vi "Robot Global Data.vi"() -> ()   [LabVIEW 2019]
doc: "This global VI can contain as many global variables as you need. Place a control on the panel, give it a good name. To read or write to it from a VI, drag the icon to the diagram of that VI. You can also drag from the project. Click on the node to change which global you access. You shouldn't have multiple locations writing to a global or it will cause a race-condition."
uses:
  <vilib>/Rock Robotics/WPI/Camera/WPI_CameraImageSize.ctl
  <vilib>/Rock Robotics/WPI/DriverStation/WPI_DriverStationRobotMode2.ctl
panel:
  out "Winch Speed":dbl
  in  "Winch":bool
  in  "OC_Winch":bool
  out "Flywheel Position":dbl
  out "Turret Type":string
  out "Turret Swiv Position":dbl
  out "Flywheel 2 Velocity":dbl
  out "Flywheel 1 Velocity":dbl
  in  "Elevator Allowed":bool
  out "Turret Pos":dbl
  out "Brake Climb":bool
  out "OC_Turret Zero":bool
  in  "Required Flywheel Speed":dbl
  out "Flywheel Speed":dbl
  out "Flywheels":bool
  out "OC_Flywheels On":bool
  out "OC_Flywheels Off":bool
  out "Fire":bool
  out "OC_Fire":bool
  in  "Turret Semi":bool
  out "OC_Turret Semi":bool
  in  "Ball Taken":bool
  out "Tower Feed On":bool
  out "Cell Counter":dbl
  in  "Tower Auto":bool
  out "OC_Tower Auto":bool
  in  "Man Tower Feed":bool
  out "OC_Man Tower Feed":bool
  out "Tower LS On":bool
  in  "Zoom In":bool
  out "OC_Lime Zoom":bool
  out "VP On":bool
  out "OC_VP Off":bool
  out "OC_VP On":bool
  out "Shooter Feed On":bool
  out "OC_Shooter Feed":bool
  out "OC_Tower Unjam":bool
  in  "Tower Unjam":bool
  out "Shooter Feed":dbl
  out "Tower Storage":dbl
  out "Tower Feed":dbl
  out "Turret Vert Value":dbl
  in  "Intake Unjam":bool
  out "DC_Intake Unjam":bool
  out "Intake Speed":dbl
  out "DC_Intake Off":bool
  out "DC_Intake On":bool
  out "DC_Intake Down":bool
  in  "Manual High":bool
  in  "DC_Manual Shift":bool
  out "Target Distance":dbl
  in  "Turret Tilted Up":bool
  out "Manual Roller":dbl
  in  "Intake Down":bool
  out "Manual Swivel Speed":dbl
  out "DC_Shifting":bool
  in  "Automatic Shift":bool
  in  "A Drv":bool
  out "High Gear":bool
  in  "Turret Manual":bool
  in  "Turret Auto":bool
  out "OC_Turret Manual":bool
  out "OC_Turret Auto":bool
  in  "Autonomous Protocol":dbl
  out "A_State":dbl
  out "Turret Up":bool
  out "OC_Turret Vert":dbl
  out "ORCA Brake":bool
  out "OC_ORCA Brake":bool
  out "Shift Storage":bool
  out "OC_Shift Storage":bool
  out "WOF Abort":bool
  out "ORCA Wheels Man":dbl
  out "Elevator":dbl
  out "OC_ORCA V Man":dbl
  out "OC_ORCA H Man":dbl
  out "DC_WOF Abort":bool
  out "WOF Pos":bool
  out "DC_WOF Pos":bool
  out "Challenge Color":string
  out "Turret Swiv Speed":dbl
  out "OC_Turret Swivel":dbl
  out "Turret Speed":dbl
  in  "Turret On":bool
  out "OC_Turret":dbl
  out "Roller Speed":dbl
  in  "Intake On":bool
  out "SC_Grab Cell":bool
  out "A ORCA Wheels":dbl
  out "ORCA Align":bool
  out "OC_ORCA Align":bool
  out "Orca Z":dbl
  out "Orca Y":dbl
  out "Orca X":dbl
  out "DC_WOF":bool
  out "WOF Limit":bool
  out "Auto Color Detected":string
  out "WOF Auto":bool
  out "Color Counter":dbl
  out "Color":string
  in  "OC_Rumble":bool
  in  "DC_Lime Cam":bool
  in  "DC_Gyro-R":bool
  out "Drv Input 2":dbl
  out "Drv Input 1":dbl
  in  "DC_Auto R TS":bool
  in  "DC_Search":bool
  in  "DC_Halo On":bool
  in  "DC_Exit VP":bool
  in  "DC_Reverse":bool
  in  "DC_Precision":bool
  out "A Drv-R":dbl
  out "A Drv-L":dbl
  out "PC6":dbl
  out "PC5":dbl
  out "PC4":dbl
  out "PC3":dbl
  out "PC2":dbl
  out "PC1":dbl
  out "LC8":dbl
  out "LC7":dbl
  out "LC6":dbl
  out "LC5":dbl
  out "LC4":dbl
  out "LC3":dbl
  out "LC2":dbl
  out "LC1":dbl
  in  "FP":bool
  out "CLS cal":dbl
  in  "Gyro Reset":bool
  out "G Offset":dbl
  out "G Cal":dbl
  out "Z-Axis":dbl format="%.2f"
  out "Y-Axis":dbl format="%.2f"
  out "X-Axis":dbl format="%.2f"
  out "Gyro":dbl
  in  "Exit VP":bool
  in  "Lime Cam":bool
  in  "D_Enc-R":bool
  out "Drift Cal":dbl
  out "Turn Cal":dbl
  in  "Locked On":bool
  in  "Tracking":bool
  in  "A Exit":bool
  in  "Drv Spd Av":dbl(knob) scale=-30.0..30.0
  out "Drv Dist Av":dbl
  out "Drv Dist R":dbl format="%.2f"
  out "Drv Spd R":dbl format="%.2f"
  out "Drv Dist L":dbl format="%.2f"
  out "Drv Spd L":dbl format="%.2f"
  in  "Centering TS":bool
  in  "Halo On":bool
  in  "Reverse":bool
  in  "Precision":bool
  in  "Drv-R-Out":dbl(knob) scale=-1.0..1.0
  in  "Drv-L-Out":dbl(knob) scale=1.0..-1.0
  out "Drive":string(combo)="Cheesy"
  out "D_Buttons":T1
  out "O2_Buttons":T1
  out "O2_Axis":T2
  out "O1_Axis":T2
  out "D_Axis":T2
  out "O1_Buttons":T1
  out "O2_POV":dbl
  out "O1_POV":dbl
  out "D_POV":dbl
  out "Y Val":dbl
  out "M Val":dbl
  out "C Val":dbl
  out "VP Select":string(combo)="XBox"
  in  "Dash In View":bool
  in  "Lime In View":bool
  in  "VP In View":bool
  out "VP X":dbl(knob) scale=-150.0..150.0
  out "Lime X":dbl
  in  "Snapshot":bool
  out "Dash X":dbl
  out "Stream":i8
  out "CamMode":i8
  out "LedMode":i8
  in  "Robot Lights":i8
  out "Light Temp":i8
  in  "Rumble":bool
  out "Rumble Time":dbl
  out "Light Select":i8
  out "O_Controller":string(combo)="XBox"
  out "D_Controller":string(combo)="XBox"
  in  "U Button":bool
  in  "LED 9":bool
  in  "LED 8":bool
  in  "LED 7":bool
  in  "LED 6":bool
  in  "LED 5":bool
  in  "LED 3":bool
  in  "LED 4":bool
  in  "LED 1":bool
  in  "LED 2":bool
  out "Match T":dbl
  out "Game Data":string
  out "Tele Time":dbl
  in  "Robot Mode 3":T3
  in  "image size 2":T4=enum."320x240"
  in  "Enable Vision 2":bool=TRUE
  out "V06":dbl
  out "V08":dbl
  out "V00":dbl
  out "V11":dbl
  out "Key Pressed":T5(array[ring])
  out "Key Enum":i16
  out "V10":dbl
  out "V09":dbl
  out "Auto R":i8
  out "Dash Select":i8
  out "V07":dbl
  out "V05":dbl
  out "V04":dbl
  out "V03":dbl
  out "V02":dbl
  out "V01":dbl
  in  "Robot Mode":T3
  in  "image size":T4=enum."320x240"
  in  "Enable Vision":bool
  # "Dashboard"
  # "External Controls"
  # "User Controls"
  # "Vision Processing"
  # "Controller Variables"
  # "Quick variable binding"
  # "Dash Array"
  # "Diagnostics"
  # "Driver Functions"
  # "Operator Functions"
  # "Operator Control Variables"
  # "Driver Control Variables"
  # "Gyro"
  # "Accelerometer"
  # "Autonomous Variables"
  # "Shared Control Variables"
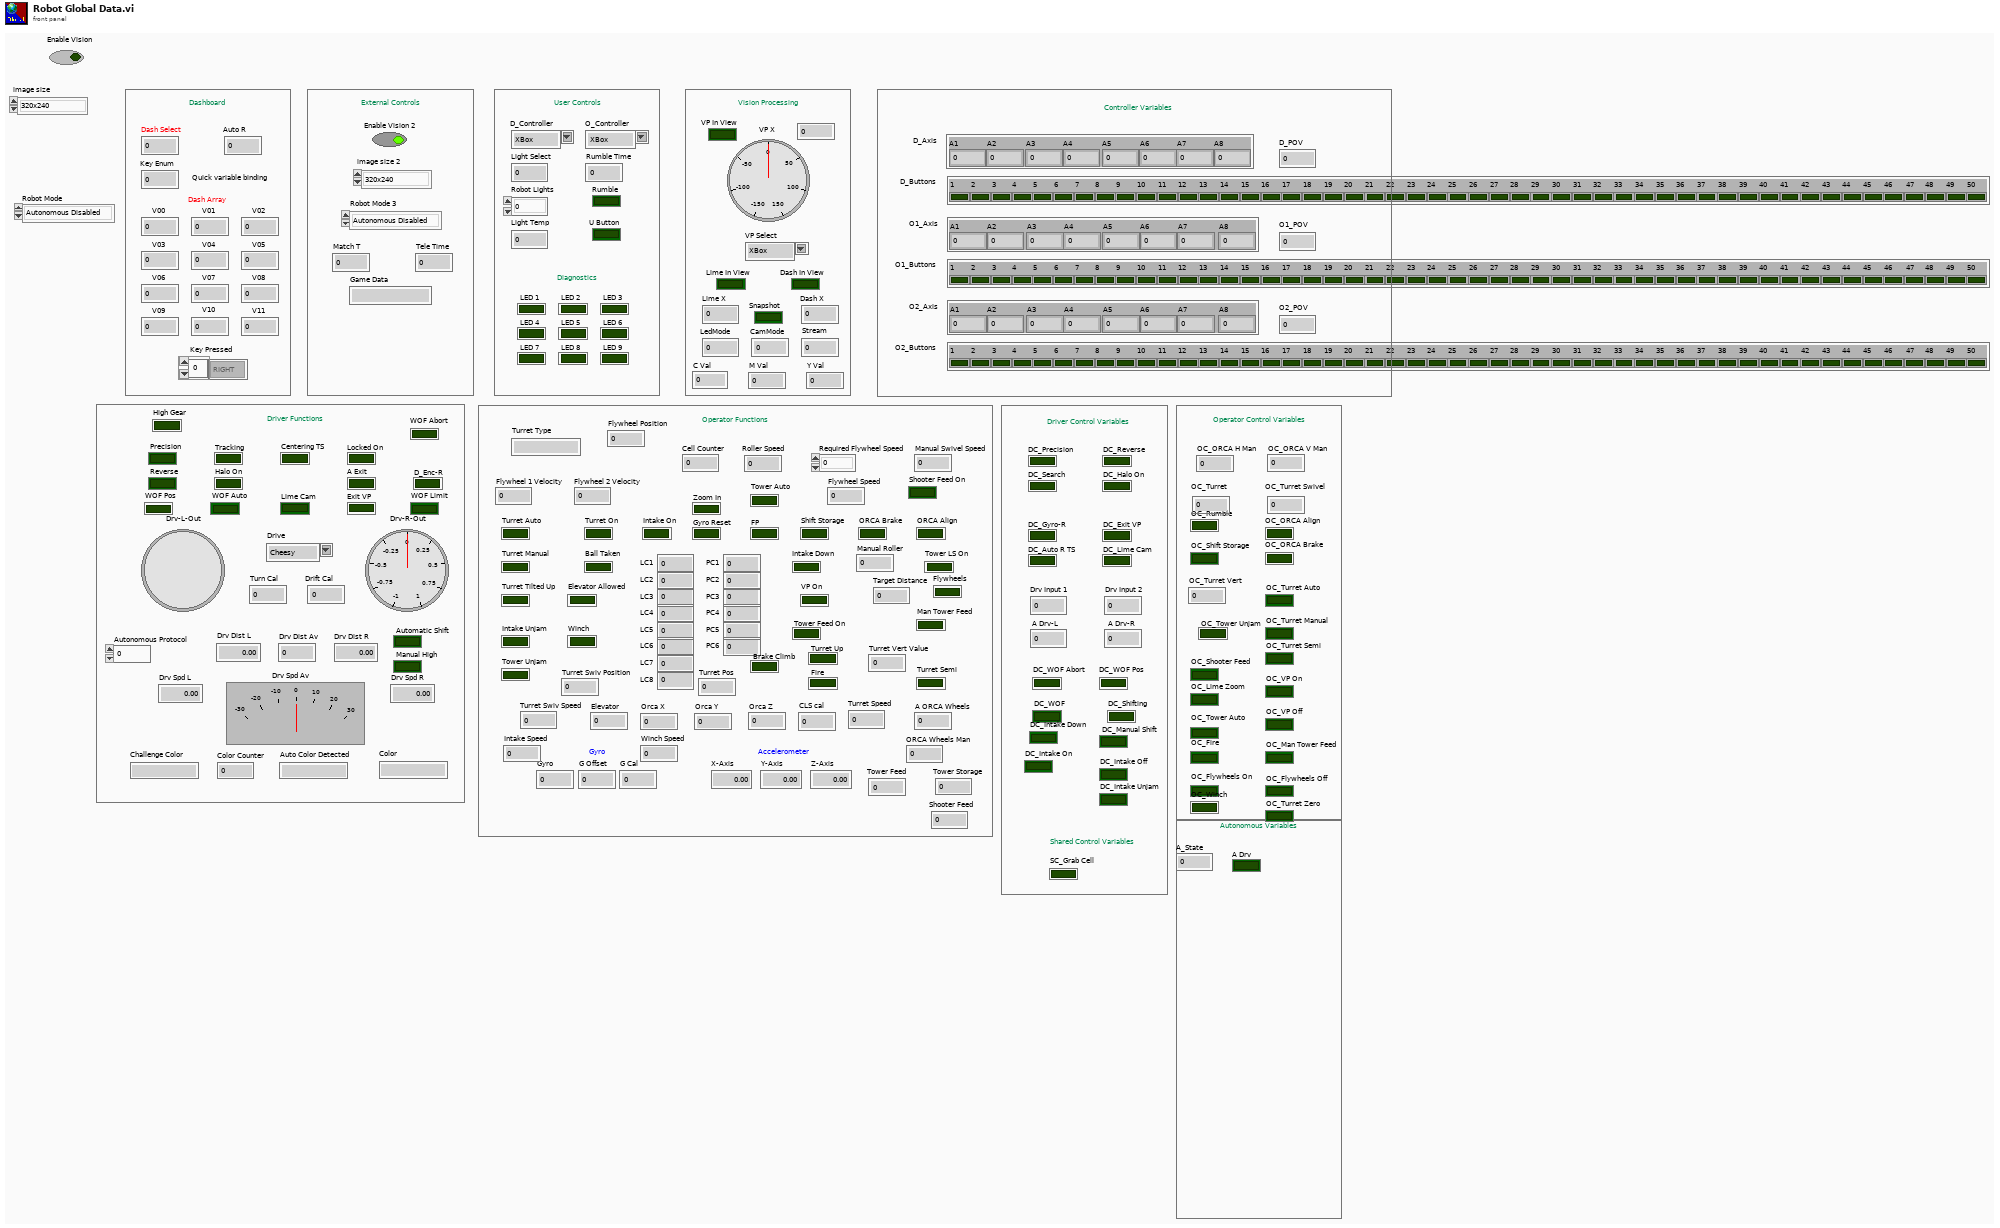
[diagram p1: front panel]
types:
  T1 = cluster{"1":bool, "2":bool, "3":bool, "4":bool, "5":bool, "6":bool, "7":bool, "8":bool, "9":bool, "10":bool, "11":bool, "12":bool, "13":bool, "14":bool, "15":bool, "16":bool, "17":bool, "18":bool, "19":bool, "20":bool, "21":bool, "22":bool, "23":bool, "24":bool, "25":bool, "26":bool, "27":bool, "28":bool, "29":bool, "30":bool, "31":bool, "32":bool, "33":bool, "34":bool, "35":bool, "36":bool, "37":bool, "38":bool, "39":bool, "40":bool, "41":bool, "42":bool, "43":bool, "44":bool, "45":bool, "46":bool, "47":bool, "48":bool, "49":bool, "50":bool}
  T2 = cluster{"A1":dbl, "A2":dbl, "A3":dbl, "A4":dbl, "A5":dbl, "A6":dbl, "A7":dbl, "A8":dbl}
  T3 = typedef "WPI_DriverStationRobotMode2.ctl" = enum16{"Autonomous Disabled", "Autonomous Enabled", "Teleop Disabled", "Teleop Enabled", "Disconnected", "Finish", "Test Disabled", "Test Enabled", "Emergency Stopped"}
  T4 = typedef "WPI_CameraImageSize.ctl" = enum16{"640x480", "320x240", "160x120", "Custom"}
  T5 = enum16{"0", "1", "2", "3", "4", "5", "6", "7", "8", "9", "A", "B", "C", "D", "E", "F", "G", "H", "I", "J", "K", "L", "M", "N", "O", "P", "Q", "R", "S", "T", "U", "V", "W", "X", "Y", "Z", "F1", "F2", "F3", "F4", "F5", "F6", "F7", "F8", "F9", "F10", "F11", "F12", "F13", "F14", "F15", "ADD", "BACK", "BACKSLASH", "CAPITAL", "COMMA", "DECIMAL", "DELETE", "DIVIDE", "DOWN", "END", "EQUALS", "ESCAPE", "GRAVE (`)", "HOME", "INSERT", "LBRACKET", "LCONTROL", "LEFT", "L ALT", "LSHIFT", "LWIN", "MINUS", "MULTIPLY", "NEXT", "NUMLOCK", "NUMPAD_0", "NUMPAD_1", "NUMPAD_2", "NUMPAD_3", "NUMPAD_4", "NUMPAD_5", "NUMPAD_6", "NUMPAD_7", "NUMPAD_8", "NUMPAD_9", "PAUSE", "PERIOD", "PRIOR (PG UP)", "RBRACKET", "RCONTROL", "RETURN", "RIGHT", "R ALT", "RSHIFT", "RWIN", "SCROLL", "SEMICOLON", "SLASH", "SPACE", "SUBTRACT", "TAB", "UP", "ENTER (num pad)", "' (quote)"}[]
diagram:
